vi "GenerateArmMotionProfilePoints.vi"(3 "MotionProfileGeneratorParameters":T4={"Trajectory Point Interval (ms)"=10, "Maximum Travel Speed (units/s)"=0.0, "Velocity Ramp Time (ms)"=0.0, "Acceleration Ramp Time (ms)"=1.0} {"Acceleration Ramp Time (ms)" min=1.0; "Velocity Ramp Time (ms)" min=1.0; "Maximum Travel Speed (units/s)" min=0.0; "Trajectory Point Interval (ms)" items=["TrajectoryDuration_0ms"=0, "TrajectoryDuration_5ms"=5, "TrajectoryDuration_10ms"=10, "TrajectoryDuration_20ms"=20, "TrajectoryDuration_30ms"=30, "TrajectoryDuration_40ms"=40, "TrajectoryDuration_50ms"=50, "TrajectoryDuration_100ms"=100]}, 4 "PathDistance":dbl, 5 "ArmPathIn":T1[](array[typedef]), 6 "IndexedPathLength":dbl[](array[numeric])) -> (0 "ArmPathOut":T1[](array[typedef]), 1 "ExtendPath":T2[](array[typedef]) {"Time (ms)" items=["TrajectoryDuration_0ms"=0, "TrajectoryDuration_5ms"=5, "TrajectoryDuration_10ms"=10, "TrajectoryDuration_20ms"=20, "TrajectoryDuration_30ms"=30, "TrajectoryDuration_40ms"=40, "TrajectoryDuration_50ms"=50, "TrajectoryDuration_100ms"=100]}, 2 "RotatePath":T2[](array[typedef]) {"Time (ms)" items=["TrajectoryDuration_0ms"=0, "TrajectoryDuration_5ms"=5, "TrajectoryDuration_10ms"=10, "TrajectoryDuration_20ms"=20, "TrajectoryDuration_30ms"=30, "TrajectoryDuration_40ms"=40, "TrajectoryDuration_50ms"=50, "TrajectoryDuration_100ms"=100]})   [LabVIEW 2017]
uses:
  TypeDefs/ArmCoordinate.ctl
  General/MotionProfiling/TypeDefs/MotionProfileGeneratorParams.ctl
  <vilib>/Rock Robotics/WPI/ThirdParty/Phoenix-LabVIEW/Motor Controller/Controls/CTRE_Phoenix_MotorControl_TrajectoryPointTimeDur.ctl
  General/MotionProfiling/TypeDefs/TrajectoryPoint.ctl
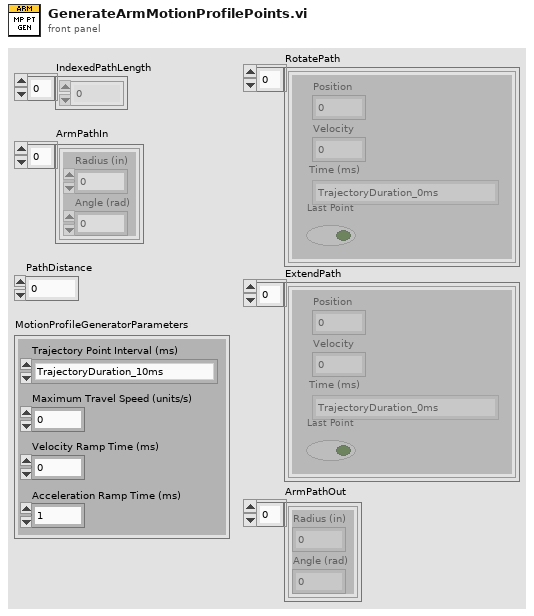
[diagram p1: front panel]
types:
  T1 = typedef "ArmCoordinate.ctl" = cluster{"Radius (in)":dbl, "Angle (rad)":dbl}
  T2 = typedef "TrajectoryPoint.ctl" = cluster{"Position ":dbl, "Velocity ":dbl, "Time (ms)":T3, "Last Point":bool}
  T3 = typedef "CTRE_Phoenix_MotorControl_TrajectoryPointTimeDur.ctl" = i32
  T4 = typedef "MotionProfileGeneratorParams.ctl" = cluster{"Trajectory Point Interval (ms)":T3, "Maximum Travel Speed (units/s)":dbl, "Velocity Ramp Time (ms)":dbl, "Acceleration Ramp Time (ms)":dbl}
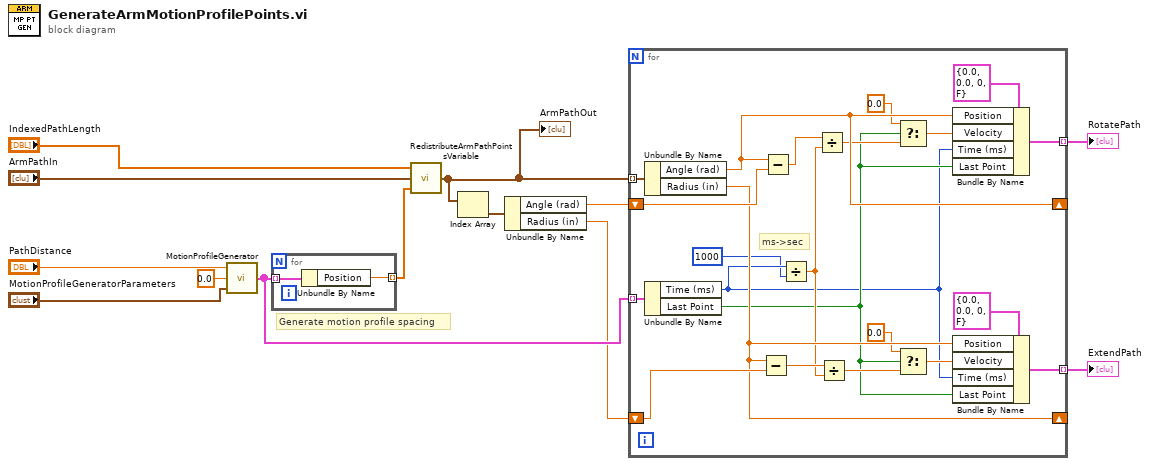
[diagram p0: block diagram]
diagram:
  # "Generate motion profile spacing"
  n1 = call "MotionProfileGenerator.vi"("MotionProfileGeneratorParameters"="MotionProfileGeneratorParameters", "Starting Position (units)"=0.0 ("Starting Position (rotations)"), "Travel Distance (units)"="PathDistance") -> ("Trajectory Points"=w3:T2[])
  n2 = for {
    tunnel: w3 -> [w15] mode=indexing
    tunnel: [w14] -> w12 mode=indexing
    n3 = Unbundle By Name(w15) -> ("Position"=w14:dbl)
  }
  n4 = call "RedistributeArmPathPointsVariable.vi"("DesiredPointSpacing"=w12, "ArmPathIn"="ArmPathIn", "IndexedPathLength"="IndexedPathLength") -> ("ArmPathOut"=w5:T1[])
  "ArmPathOut" <- w5
  n5 = Index Array(array=w5) -> (element=w4:T1)  [unwired: 1 in]
  n6 = Unbundle By Name(w4) -> ("Angle (rad)"=w2:dbl, "Radius (in)"=w1:dbl)
  n7 = for {
    tunnel: w5 -> [w32] mode=indexing
    tunnel: w3 -> [w33] mode=indexing
    tunnel: [w35] -> w6 mode=indexing
    tunnel: [w34] -> w7 mode=indexing
    shift-right: [w30] -> _
    shift-left: w2 -> [w31]
    shift-right: [w28] -> _
    shift-left: w1 -> [w29]
    # "ms->sec"
    n8 = Unbundle By Name(w32) -> ("Angle (rad)"=w30:dbl, "Radius (in)"=w28:dbl)
    n9 = Unbundle By Name(w33) -> ("Time (ms)"=w17:T3, "Last Point"=w20:bool)
    n10 = Subtract(x=w28, y=w29) -> (x-y=w27:dbl)
    n11 = Subtract(x=w30, y=w31) -> (x-y=w26:dbl)
    n12 = Divide(x=w17, y=1000) -> (x/y=w25:dbl)
    n13 = Divide(x=w26, y=w25) -> (x/y=w24:dbl)
    n14 = Divide(x=w27, y=w25) -> (x/y=w21:dbl)
    n15 = Select(t=0.0, s=w20, f=w24) -> (s? t:f=w23:dbl)
    n16 = Select(t=0.0, s=w20, f=w21) -> (s? t:f=w19:dbl)
    n17 = Bundle By Name(cluster=T2 {"Position "=0.0, "Velocity "=0.0, "Time (ms)"=0, "Last Point"=FALSE} ("trajectory point"), "Position"=w30, "Velocity"=w23, "Time (ms)"=w17, "Last Point"=w20) -> (w34:T2)
    n18 = Bundle By Name(cluster=T2 {"Position "=0.0, "Velocity "=0.0, "Time (ms)"=0, "Last Point"=FALSE} ("trajectory point"), "Position"=w28, "Velocity"=w19, "Time (ms)"=w17, "Last Point"=w20) -> (w35:T2)
  }
  "RotatePath" <- w7
  "ExtendPath" <- w6
